vi "Sort 2D Array (CXT)__ogtk.vi"(6 "Column/Row to Sort By":u32, 7 "Method (magnitude)":enum16{"real", "imaginary", "magnitude"}(ring)=enum."magnitude", 8 "Sort By in":enum16{"row", "column"}(ring), 9 "Order":enum16{"ascending", "descending"}(ring), 11 "Array in":cxt[][](array[numeric]) format="%.2f") -> (0 "Sort By out":enum16{"row", "column"}(ring), 1 "Index Out of Range?":bool, 2 "Sorted Pointers":i32[](array[numeric]), 3 "Sorted Array out":cxt[][](array[numeric]) format="%.2f")   [LabVIEW 2020]
doc: "This polymorphic VI sorts a 2D array of numerics or strings, regardless of the array size. You can specify whether to sort by column or row, which column or row to sort by, and whether to sort in ascending or descending order. You also can specify a secondary row or column to sort by."
panel:
  # "Sort 2D Array\n\nThis VI sorts by row or by column, a 2D array of any size in descending or ascending order based on a column or row whose index you specify.\n\nPlease visit http://www.OpenG.org to learn about the\nOpen Source LabVIEW software movement.\n\nNOTICE -- YOU MUST LEAVE THIS NOTICE IN PLACE.  PER THE TERMS OF THE LICENSE BELOW, YOU MAY SUBLICENSE THIS SOFTWARE \nIN ANY WAY THAT DOES NOT CONFLICT WITH THIS LICENSE.\n\n### BSD License (http://www.opensource.org/licenses/bsd-license.php) Begin ###\n \nCopyright (c) 2002, Jim Kring <jim@jimkring.com>\nCopyright (c) 2002, Cal-Bay Systems, Inc. <info@calbay.com>\n\nAll rights reserved.\n\nRedistribution and use in source and binary forms, with or without modification, are permitted provided that the following conditions are met:\n\n    * Redistributions of source code must retain the above copyright notice, this list of conditions and the following disclaimer.\n    * Redistributions in binary form must reproduce the above copyright notice, this list of conditions and the following disclaimer in the \n       documentation and/or other materials provided with the distribution.\n    * Neither the name of SciWare, James Kring, Inc., nor the names of its contributors may be used to endorse or promote products derived \n       from this software without specific prior written permission.\n\nTHIS SOFTWARE IS PROVIDED BY THE COPYRIGHT HOLDERS AND CONTRIBUTORS \"AS IS\" AND ANY EXPRESS OR IMPLIED WARRANTIES, \nINCLUDING, BUT NOT LIMITED TO, THE IMPLIED WARRANTIES OF MERCHANTABILITY AND FITNESS FOR A PARTICULAR PURPOSE ARE \nDISCLAIMED. IN NO EVENT SHALL THE COPYRIGHT OWNER OR CONTRIBUTORS BE LIABLE FOR ANY DIRECT, INDIRECT, INCIDENTAL,\n SPECIAL, EXEMPLARY, OR CONSEQUENTIAL DAMAGES (INCLUDING, BUT NOT LIMITED TO, PROCUREMENT OF SUBSTITUTE GOODS OR \nSERVICES; LOSS OF USE, DATA, OR PROFITS; OR BUSINESS INTERRUPTION) HOWEVER CAUSED AND ON ANY THEORY OF LIABILITY, \nWHETHER IN CONTRACT, STRICT LIABILITY, OR TORT (INCLUDING NEGLIGENCE OR OTHERWISE) ARISING IN ANY WAY OUT OF THE USE \nOF THIS SOFTWARE, EVEN IF ADVISED OF THE POSSIBILITY OF SUCH DAMAGE.\n\n### BSD License End ###"
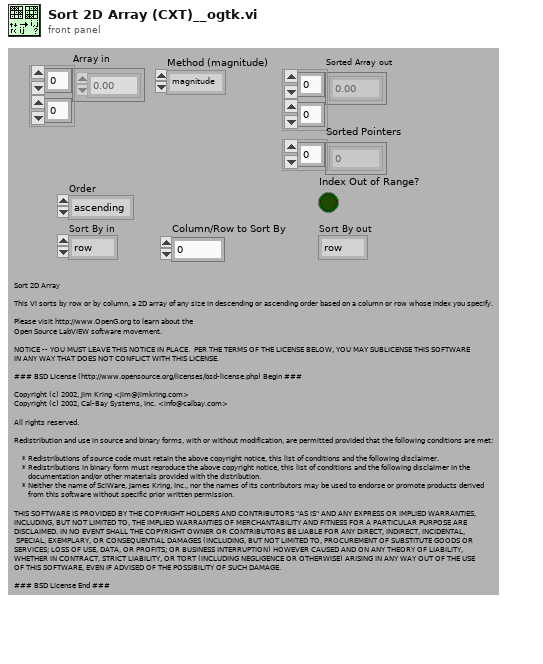
[diagram p1: front panel]
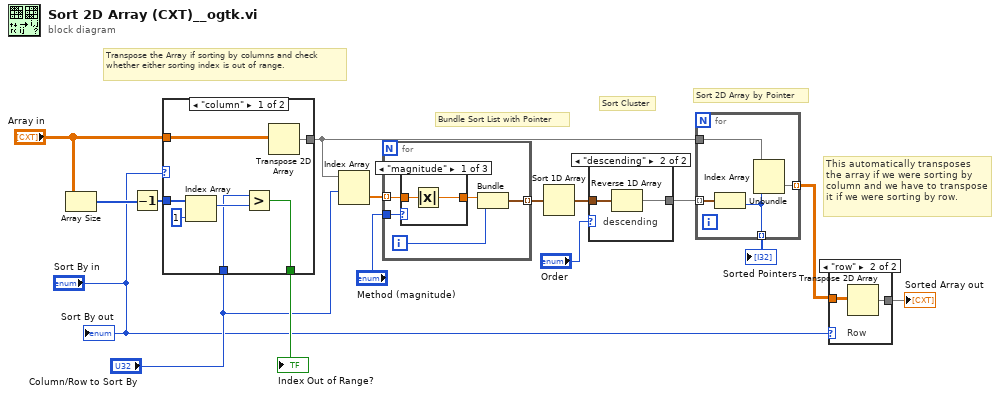
[diagram p0: block diagram]
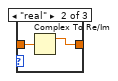
[diagram p2: hidden frame]
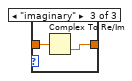
[diagram p3: hidden frame]
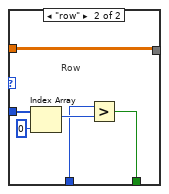
[diagram p6: hidden frame]
diagram:
  # "Sort 2D Array by Pointer"
  # "Sort Cluster"
  # "This automatically transposes the array if we were sorting by column and we have to transpose it if we were sorting by row."
  # "Bundle Sort List with Pointer"
  # "Transpose the Array if sorting by columns and check whether either sorting index is out of range."
  n1 = Array Size(array="Array in") -> (size(s)=w12:i32[])
  n2 = Decrement(x=w12) -> (x-1=w9:i32[])
  n3 = case shown="\"column\"" "Sort By in" {
    tunnel: "Array in" -> [w23 w29]
    tunnel: [w22 w29] -> w16
    tunnel: w9 -> [w21 w26]
    tunnel: [w17 w24] -> w11
    tunnel: "Column/Row to Sort By" -> [w18 w25]
    frame "column" {
      n4 = Index Array(array=w21, index=1 ("Index")) -> (element=w19:i32)
      n5 = Greater?(x=w18, y=w19) -> (0:w17:bool)
      n6 = Transpose 2D Array(2D array=w23) -> (transposed array=w22:cxt[][])
    }
    frame "row" {
      # "Row"
      n7 = Index Array(array=w26, index=0 ("Index")) -> (element=w28:i32)
      n8 = Greater?(x=w25, y=w28) -> (0:w24:bool)
    }
  }
  "Index Out of Range?" <- w11
  n9 = Index Array(array=w16, index (row)="Column/Row to Sort By") -> (element=w3:cxt[])  [unwired: 1 in]
  n10 = for {
    tunnel: w3 -> [w33] mode=indexing
    tunnel: [w34] -> w2 mode=indexing
    tunnel: "Method (magnitude)" -> [w30]
    i -> [w31]
    n11 = case shown="\"magnitude\"" w30 {
      tunnel: w33 -> [w36 w38 w40]
      tunnel: [w35 w37 w39] -> w32
      frame "magnitude" {
        n12 = Absolute Value(x=w36) -> (abs(x)=w35:ext)
      }
      frame "real" {
        n13 = Complex To Re/Im(x + iy=w38) -> (x=w37:ext)  [unwired: 1 out]
      }
      frame "imaginary" {
        n14 = Complex To Re/Im(x + iy=w40) -> (y=w39:ext)  [unwired: 1 out]
      }
    }
    n15 = Bundle(w32, w31) -> (w34:cluster{ext, i32})  [unwired: 1 in]
  }
  n16 = Sort 1D Array(array=w2) -> (sorted array=w6:cluster{ext, i32}[])
  n17 = case shown="\"descending\"" "Order" {
    tunnel: [w41 w42] -> w7
    tunnel: w6 -> [w41 w43]
    frame "ascending", Default {
    }
    frame "descending" {
      # "descending"
      n18 = Reverse 1D Array(array=w43) -> (reversed array=w42:cluster{ext, i32}[])
    }
  }
  n19 = for {
    tunnel: w7 -> [w47] mode=indexing
    tunnel: w16 -> [w46]
    tunnel: [w45] -> w15 mode=indexing
    tunnel: [w44] -> w5 mode=indexing
    n20 = Unbundle(w47) -> (w44:i32)  [unwired: 1 out]
    n21 = Index Array(array=w46, index (col)=w44) -> (element=w45:cxt[])  [unwired: 1 in]
  }
  "Sorted Pointers" <- w5
  n22 = case shown="\"row\"" "Sort By in" {
    tunnel: w15 -> [w48 w50]
    tunnel: [w48 w49] -> w14
    frame "column" {
    }
    frame "row" {
      # "Row"
      n23 = Transpose 2D Array(2D array=w50) -> (transposed array=w49:cxt[][])
    }
  }
  "Sorted Array out" <- w14
  "Sort By out" <- "Sort By in"
